vi "Lab Panel V4.85.vi"() -> ()   [LabVIEW 2013] (continued)
          n209 = property on="Tab Control 2" class="TabCtl (strict)"("DisabledEnum"=T14."Enabled" ("Disabled")) -> ()  [unwired: 2 in, 2 out]
          n210 = property on="Tab Control 2" class="TabCtl (strict)"("Value"=0) -> ()  [unwired: 2 in, 2 out]
        }
        frame #9 {
          # "check network directory valid"
          n211 = while {
            stop <- w259 continue-if-true
            w257 = TRUE
            n212 = local read "Network Directory"() -> (w261:path)
            n213 = property on="Tab Control 2" class="TabCtl (strict)"("Value"=5) -> ()  [unwired: 2 in, 2 out]
            n214 = File/Directory Info(path=w261) -> (error out=w262:errorcluster)  [unwired: 1 in, 6 out]
            n215 = Unbundle(w262) -> ("status"=w259:bool)  [unwired: 2 out]
            n216 = case shown="True" w259 {
              frame False {
                n217 = local write "Message"("") -> ()
              }
              frame True {
                "Message" <- "NETWORK DIRECTORY NOT FOUND!!!!"
              }
            }
            n218 = property on="Message" class="Str"("Text.TextColor"=u32 16711680) -> ()  [unwired: 2 in, 2 out]
            n219 = property on="Network Directory" class="Path"("Blinking"=w257) -> ()  [unwired: 2 in, 2 out]
            n220 = property on="Message" class="Str"("Blinking"=w257) -> ()  [unwired: 2 in, 2 out]
          }
        }
        frame #10 {
          w265 = FALSE
          n221 = property on="Message" class="Str"("Blinking"=w265) -> ()  [unwired: 2 in, 2 out]
          n222 = property on="Network Directory" class="Path"("Blinking"=w265) -> ()  [unwired: 2 in, 2 out]
          n223 = property on="Tab Control 2" class="TabCtl (strict)"("Value"=0) -> ()  [unwired: 2 in, 2 out]
        }
      }
    }
    frame #2 {
      n224 = node-c288("loop  delay(mS)") -> (w269:T15)  [unwired: 3 in]
      n225 = timed-loop {
        timing: w269 -> [_]
        timing-out: [_] -> w268
        i -> [w291]
        stop <- "stop" stop-if-true
        n226 = node-c288() -> ()  [unwired: 1 in, 1 out]
        n227 = global write "Global display 1.vi" "stop disp"("stop") -> ()
        n228 = local read "SELECT LAB05-2"() -> (w271:T3)
        n229 = local read "SELECT LAB05-1"() -> (w272:T3)
        n230 = local read "SELECT LAB04-2"() -> (w273:T3)
        n231 = local read "SELECT LAB03-1"() -> (w276:T3)
        n232 = local read "SELECT LAB02-2"() -> (w277:T3)
        n233 = local read "SELECT LAB01-1"() -> (w280:T3)
        n234 = local read "SELECT LAB03-2"() -> (w275:T3)
        n235 = local read "SELECT LAB01-2"() -> (w279:T3)
        n236 = local read "SELECT LAB04-1"() -> (w274:T3)
        n237 = local read "SELECT LAB02-1"() -> (w278:T3)
        n238 = local read "run lab03-2"() -> (w285:bool)
        n239 = local read "run lab04-1"() -> (w284:bool)
        n240 = local read "run lab05-1"() -> (w282:bool)
        n241 = local read "run lab04-2"() -> (w283:bool)
        n242 = local read "run lab05-2"() -> (w281:bool)
        n243 = local read "run lab03-1"() -> (w286:bool)
        n244 = local read "run lab02-2"() -> (w287:bool)
        n245 = local read "run lab02-1"() -> (w288:bool)
        n246 = local read "run lab01-1"() -> (w290:bool)
        n247 = local read "run lab01-2"() -> (w289:bool)
        n248 = stacked-sequence {
          seq-local: [_ w353 _ _ _ _ _ _ _ _ _ _ _ _ _ _ _ _ _ _ _ _] -> [_ _ _ _ _ w2145 _ _ _ _ _ _ _ _ _ _ _ _ _ _ _ _]
          seq-local: [_ w352 _ _ _ _ _ _ _ _ _ _ _ _ _ _ _ _ _ _ _ _] -> [_ _ _ _ _ w2144 _ _ _ _ _ _ _ _ _ _ _ _ _ _ _ _]
          seq-local: [_ w339 _ _ _ _ _ _ _ _ _ _ _ _ _ _ _ _ _ _ _ _] -> [_ _ _ _ _ w2143 _ _ _ _ _ _ _ _ _ _ _ _ _ _ _ _]
          seq-local: [_ w338 _ _ _ _ _ _ _ _ _ _ _ _ _ _ _ _ _ _ _ _] -> [_ _ _ _ _ w2142 _ _ _ _ _ _ _ _ _ _ _ _ _ _ _ _]
          seq-local: [_ w337 _ _ _ _ _ _ _ _ _ _ _ _ _ _ _ _ _ _ _ _] -> [_ _ _ _ _ w2141 _ _ _ _ _ _ _ _ _ _ _ _ _ _ _ _]
          seq-local: [_ w336 _ _ _ _ _ _ _ _ _ _ _ _ _ _ _ _ _ _ _ _] -> [_ _ _ _ _ w2140 _ _ _ _ _ _ _ _ _ _ _ _ _ _ _ _]
          seq-local: [_ w335 _ _ _ _ _ _ _ _ _ _ _ _ _ _ _ _ _ _ _ _] -> [_ _ _ _ _ w2139 _ _ _ _ _ _ _ _ _ _ _ _ _ _ _ _]
          seq-local: [_ w334 _ _ _ _ _ _ _ _ _ _ _ _ _ _ _ _ _ _ _ _] -> [_ _ _ _ _ w2138 _ _ _ _ _ _ _ _ _ _ _ _ _ _ _ _]
          seq-local: [_ w333 _ _ _ _ _ _ _ _ _ _ _ _ _ _ _ _ _ _ _ _] -> [_ _ _ _ _ w2137 _ _ _ _ _ _ _ _ _ _ _ _ _ _ _ _]
          seq-local: [_ w332 _ _ _ _ _ _ _ _ _ _ _ _ _ _ _ _ _ _ _ _] -> [_ _ _ _ _ w2136 _ _ _ _ _ _ _ _ _ _ _ _ _ _ _ _]
          tunnel: w290 -> [_ _ w369 w611 w1735 w2165 w2480 w2967 _ _ _ _ w3371 _ w4305 _ _ w4590 w4893 w5074 _ _]
          tunnel: w289 -> [_ _ w368 w609 w1734 w2164 w2481 w2966 _ _ _ _ w3370 _ w4303 _ _ w4589 w4892 w5072 _ _]
          tunnel: w288 -> [_ _ w367 w607 w1733 w2163 w2479 w2965 _ _ _ _ w3369 _ w4301 _ _ w4588 w4891 w5071 _ _]
          tunnel: w287 -> [_ _ w366 w605 w1732 w2162 w2478 w2964 _ _ _ _ w3368 _ w4299 _ _ w4587 w4890 w5070 _ _]
          tunnel: w286 -> [_ _ w365 w603 w1731 w2161 w2477 w2963 _ _ _ _ w3367 _ w4297 _ _ w4586 w4889 w5069 _ _]
          tunnel: w285 -> [_ _ w364 w601 w1730 w2160 w2476 w2962 _ _ _ _ w3366 _ w4295 _ _ w4585 w4888 w5068 _ _]
          tunnel: w284 -> [_ _ w363 w599 w1729 w2159 w2475 w2961 _ _ _ _ w3365 _ w4293 _ _ w4584 w4887 w5067 _ _]
          tunnel: w283 -> [_ _ w362 w597 w1728 w2158 w2474 w2960 _ _ _ _ w3364 _ w4291 _ _ w4583 w4886 w5066 _ _]
          tunnel: w282 -> [_ _ w361 w595 w1727 w2157 w2473 w2959 _ _ _ _ w3363 _ w4289 _ _ w4582 w4885 w5065 _ _]
          tunnel: w281 -> [_ _ w360 w593 w1726 w2156 w2472 w2958 _ _ _ _ w3362 _ w4287 _ _ w4581 w4884 w5064 _ _]
          tunnel: w280 -> [_ _ _ w610 w1725 w2155 _ _ _ _ _ _ _ _ w4307 _ _ _ _ _ w5368 _]
          tunnel: w279 -> [_ _ _ w608 w1724 w2154 _ _ _ _ _ _ _ _ w4302 _ _ _ _ _ w5367 _]
          tunnel: w278 -> [_ _ _ w606 w1723 w2153 _ _ _ _ _ _ _ _ w4300 _ _ _ _ _ w5366 _]
          tunnel: w277 -> [_ _ _ w604 w1722 w2152 _ _ _ _ _ _ _ _ w4298 _ _ _ _ _ w5365 _]
          tunnel: w276 -> [_ _ _ w602 w1721 w2151 _ _ _ _ _ _ _ _ w4296 _ _ _ _ _ w5364 _]
          tunnel: w275 -> [_ _ _ w600 w1720 w2150 _ _ _ _ _ _ _ _ w4294 _ _ _ _ _ w5363 _]
          tunnel: w274 -> [_ _ _ w598 w1719 w2149 _ _ _ _ _ _ _ _ w4292 _ _ _ _ _ w5362 _]
          tunnel: w273 -> [_ _ _ w596 w1718 w2148 _ _ _ _ _ _ _ _ w4290 _ _ _ _ _ w5361 _]
          tunnel: w272 -> [_ _ _ w594 w1717 w2147 _ _ _ _ _ _ _ _ w4288 _ _ _ _ _ w5360 _]
          tunnel: w271 -> [_ _ _ w592 w1716 w2146 _ _ _ _ _ _ _ _ w4286 _ _ _ _ _ w5359 _]
          frame #0 {
            w295 = FALSE
            w300 = 0.5
            # "set up cycle control"
            n249 = local read "jig cycle"() -> (w299:dbl)
            n250 = Divide(x="JIG ON TIME (S)", y=w300) -> (x/y=→"on loops":dbl)
            n251 = Divide(x="JIG OFF TIME (S)", y=w300) -> (x/y=→"off loops":dbl)
            n252 = Increment(x=w299) -> (x+1=w298:dbl)
            n253 = local write "TEMP"(w295) -> ()
            n254 = local write "AI"(w295) -> ()
            n255 = local write "jig cycle"(w298) -> ()
            n256 = event shown="[1] \"ADMIN\": Value Change" {
              selector: _ -> [_ _]
              dyn-events: _ -> [_ _]
              timeout: 10 -> [_ _]
              event Timeout {
                n257 = event-data() -> ()  [unwired: 1 in, 3 out]
              }
              event "ADMIN": Value Change {
                n258 = event-data() -> ()  [unwired: 1 in, 6 out]
                n259 = stacked-sequence {
                  seq-local: [_ w304 _] -> [_ _ w305]
                  frame #0 {
                    n260 = global write "Global 1.vi" "password"("9999") -> ()
                  }
                  frame #1 {
                    n261 = call "sub vi - password 1.vi"() -> ("RESULT"=w304:bool)  [unwired: 11 in]
                  }
                  frame #2 {
                    w307 = FALSE
                    n262 = property on="Tab Control 2" class="TabCtl (strict)"() -> ("Pages"=w311:refnum<vi>[])  [unwired: 2 in, 2 out]
                    n263 = Select(t=TRUE, s=w305, f=w307) -> (s? t:f=w306:bool)
                    n264 = Index Array(array=w311, index=9) -> (element=w309:refnum<vi>)
                    n265 = property class="Page"(reference=w309, "PageVis"=w306) -> ()  [unwired: 1 in, 2 out]
                    n266 = local write "ADMIN"(w307) -> ()
                  }
                }
              }
            }
          }
          frame #1 {
            w349 = 60.0
            # "convert temperature rise minutes to cycles"
            n267 = local read "SET LAB05-2"() -> (w313:T5)
            n268 = local read "SET LAB05-1"() -> (w315:T5)
            n269 = local read "SET LAB04-2"() -> (w317:T5)
            n270 = local read "SET LAB01-1"() -> (w331:T5)
            n271 = local read "SET LAB01-2"() -> (w329:T5)
            n272 = local read "SET LAB02-2"() -> (w325:T5)
            n273 = local read "SET LAB04-1"() -> (w319:T5)
            n274 = local read "SET LAB03-1"() -> (w323:T5)
            n275 = local read "SET LAB03-2"() -> (w321:T5)
            n276 = local read "SET LAB02-1"() -> (w327:T5)
            n277 = local read "JIG OFF TIME (S)"() -> (w354:dbl)
            n278 = local read "JIG ON TIME (S)"() -> (w355:dbl)
            n279 = Unbundle(w313) -> ("T-RISE mins"=w312:dbl)  [unwired: 4 out]
            n280 = Unbundle(w315) -> ("T-RISE mins"=w314:dbl)  [unwired: 4 out]
            n281 = Unbundle(w331) -> ("T-RISE mins"=w330:dbl)  [unwired: 4 out]
            n282 = Unbundle(w317) -> ("T-RISE mins"=w316:dbl)  [unwired: 4 out]
            n283 = Unbundle(w329) -> ("T-RISE mins"=w328:dbl)  [unwired: 4 out]
            n284 = Unbundle(w327) -> ("T-RISE mins"=w326:dbl)  [unwired: 4 out]
            n285 = Unbundle(w319) -> ("T-RISE mins"=w318:dbl)  [unwired: 4 out]
            n286 = Unbundle(w325) -> ("T-RISE mins"=w324:dbl)  [unwired: 4 out]
            n287 = Unbundle(w321) -> ("T-RISE mins"=w320:dbl)  [unwired: 4 out]
            n288 = Unbundle(w323) -> ("T-RISE mins"=w322:dbl)  [unwired: 4 out]
            n289 = Add(x=w355, y=w354) -> (x+y=w348:dbl)
            n290 = Multiply(x=w349, y=w320) -> (x*y=w344:dbl)
            n291 = Multiply(x=w349, y=w318) -> (x*y=w343:dbl)
            n292 = Multiply(x=w349, y=w316) -> (x*y=w342:dbl)
            n293 = Multiply(x=w349, y=w314) -> (x*y=w341:dbl)
            n294 = Multiply(x=w349, y=w312) -> (x*y=w340:dbl)
            n295 = Multiply(x=w349, y=w328) -> (x*y=w350:dbl)
            n296 = Multiply(x=w349, y=w322) -> (x*y=w345:dbl)
            n297 = Multiply(x=w349, y=w330) -> (x*y=w351:dbl)
            n298 = Multiply(x=w349, y=w326) -> (x*y=w347:dbl)
            n299 = Multiply(x=w349, y=w324) -> (x*y=w346:dbl)
            n300 = Divide(x=w341, y=w348) -> (x/y=w333:dbl)
            n301 = Divide(x=w342, y=w348) -> (x/y=w334:dbl)
            n302 = Divide(x=w343, y=w348) -> (x/y=w335:dbl)
            n303 = Divide(x=w340, y=w348) -> (x/y=w332:dbl)
            n304 = Divide(x=w345, y=w348) -> (x/y=w337:dbl)
            n305 = Divide(x=w351, y=w348) -> (x/y=w353:dbl)
            n306 = Divide(x=w350, y=w348) -> (x/y=w352:dbl)
            n307 = Divide(x=w347, y=w348) -> (x/y=w339:dbl)
            n308 = Divide(x=w346, y=w348) -> (x/y=w338:dbl)
            n309 = Divide(x=w344, y=w348) -> (x/y=w336:dbl)
          }
          frame #2 {
            # "control cycle loops"
            n310 = local read "JIG OFF TIME (S)"() -> (w358:dbl)
            n311 = local read "JIG ON TIME (S)"() -> (w357:dbl)
            n312 = local read "jig cycle"() -> (w371:dbl)
            n313 = local read "on loops"() -> (w373:dbl)
            n314 = local read "off loops"() -> (w372:dbl)
            n315 = Add(x=w358, y=w357) -> (x+y=w356:dbl)
            n316 = Add(x=w373, y=w372) -> (x+y=w359:dbl)
            n317 = Greater Or Equal?(x=w371, y=w359) -> (x >= y?=w370:bool)
            n318 = case shown="True" w370 {
              tunnel: w369 -> [_ w408]
              tunnel: w368 -> [_ w407]
              tunnel: w367 -> [_ w406]
              tunnel: w366 -> [_ w405]
              tunnel: w365 -> [_ w404]
              tunnel: w364 -> [_ w403]
              tunnel: w363 -> [_ w402]
              tunnel: w362 -> [_ w401]
              tunnel: w361 -> [_ w400]
              tunnel: w360 -> [_ w399]
              tunnel: w356 -> [_ w398]
              frame False {
              }
              frame True {
                # "increment cycle value and convert cycles to minutes for temp rise"
                n319 = local read "Temp Loops"() -> (w375:dbl)
                n320 = local read "JIG RELAY CYCLES"() -> (w397:T7)
                n321 = Increment(x=w375) -> (x+1=w374:dbl)
                n322 = local write "Temp Loops"(w374) -> ()
                n323 = Unbundle By Name(w397) -> ("LAB01-1"=w395:dbl, "LAB01-2"=w393:dbl, "LAB02-1"=w391:dbl, "LAB02-2"=w389:dbl, "LAB03-1"=w387:dbl, "LAB03-2"=w385:dbl, "LAB04-1"=w383:dbl, "LAB04-2"=w381:dbl, "LAB05-1"=w379:dbl, "LAB05-2"=w377:dbl)
                n324 = stacked-sequence {
                  tunnel: w408 -> [w420 _ _ _ _ _ _ _ _ _]
                  tunnel: w407 -> [_ w437 _ _ _ _ _ _ _ _]
                  tunnel: w406 -> [_ _ w454 _ _ _ _ _ _ _]
                  tunnel: w405 -> [_ _ _ w471 _ _ _ _ _ _]
                  tunnel: w404 -> [_ _ _ _ w488 _ _ _ _ _]
                  tunnel: w403 -> [_ _ _ _ _ w505 _ _ _ _]
                  tunnel: w402 -> [_ _ _ _ _ _ w522 _ _ _]
                  tunnel: w401 -> [_ _ _ _ _ _ _ w539 _ _]
                  tunnel: w400 -> [_ _ _ _ _ _ _ _ w556 _]
                  tunnel: w399 -> [_ _ _ _ _ _ _ _ _ w573]
                  tunnel: w398 -> [w417 w434 w451 w468 w485 w502 w519 w536 w553 w570]
                  tunnel: w395 -> [w411 _ _ _ _ _ _ _ _ _]
                  tunnel: [w410 _ _ _ _ _ _ _ _ _] -> w394
                  tunnel: w393 -> [_ w428 _ _ _ _ _ _ _ _]
                  tunnel: [_ w427 _ _ _ _ _ _ _ _] -> w392
                  tunnel: w391 -> [_ _ w445 _ _ _ _ _ _ _]
                  tunnel: [_ _ w444 _ _ _ _ _ _ _] -> w390
                  tunnel: w389 -> [_ _ _ w462 _ _ _ _ _ _]
                  tunnel: [_ _ _ w461 _ _ _ _ _ _] -> w388
                  tunnel: w387 -> [_ _ _ _ w479 _ _ _ _ _]
                  tunnel: [_ _ _ _ w478 _ _ _ _ _] -> w386
                  tunnel: w385 -> [_ _ _ _ _ w496 _ _ _ _]
                  tunnel: [_ _ _ _ _ w495 _ _ _ _] -> w384
                  tunnel: w383 -> [_ _ _ _ _ _ w513 _ _ _]
                  tunnel: [_ _ _ _ _ _ w512 _ _ _] -> w382
                  tunnel: w381 -> [_ _ _ _ _ _ _ w530 _ _]
                  tunnel: [_ _ _ _ _ _ _ w529 _ _] -> w380
                  tunnel: w379 -> [_ _ _ _ _ _ _ _ w547 _]
                  tunnel: [_ _ _ _ _ _ _ _ w546 _] -> w378
                  tunnel: w377 -> [_ _ _ _ _ _ _ _ _ w564]
                  tunnel: [_ _ _ _ _ _ _ _ _ w563] -> w376
                  frame #0 {
                    n325 = local read "DISP LAB01-1"() -> (w415:T4)
                    n326 = Unbundle(w415) -> ("CYCLE"=w416:dbl)  [unwired: 2 out]
                    n327 = case shown="True" w420 {
                      tunnel: w416 -> [w422 w426]
                      tunnel: [w422 w425] -> w414
                      tunnel: w411 -> [w421 w424]
                      tunnel: [w421 w423] -> w410
                      frame False {
                      }
                      frame True {
                        n328 = Increment(x=w424) -> (x+1=w423:dbl)
                        n329 = Increment(x=w426) -> (x+1=w425:dbl)
                      }
                    }
                    n330 = Multiply(x=w414, y=w417) -> (x*y=w418:dbl)
                    n331 = Divide(x=w418, y=60.0) -> (x/y=w413:dbl)
                    n332 = Bundle(cluster=w415, "CYCLE"=w414, "MINS"=w413) -> (w412:T4)  [unwired: 1 in]
                    n333 = local write "DISP LAB01-1"(w412) -> ()
                  }
                  frame #1 {
                    n334 = local read "DISP LAB01-2"() -> (w432:T4)
                    n335 = Unbundle(w432) -> ("CYCLE"=w433:dbl)  [unwired: 2 out]
                    n336 = case shown="True" w437 {
                      tunnel: w433 -> [w439 w443]
                      tunnel: [w439 w442] -> w430
                      tunnel: w428 -> [w438 w441]
                      tunnel: [w438 w440] -> w427
                      frame False {
                      }
                      frame True {
                        n337 = Increment(x=w441) -> (x+1=w440:dbl)
                        n338 = Increment(x=w443) -> (x+1=w442:dbl)
                      }
                    }
                    n339 = Multiply(x=w430, y=w434) -> (x*y=w435:dbl)
                    n340 = Divide(x=w435, y=60.0) -> (x/y=w429:dbl)
                    n341 = Bundle(cluster=w432, "CYCLE"=w430, "MINS"=w429) -> (w431:T4)  [unwired: 1 in]
                    n342 = local write "DISP LAB01-2"(w431) -> ()
                  }
                  frame #2 {
                    n343 = local read "DISP LAB02-1"() -> (w449:T4)
                    n344 = Unbundle(w449) -> ("CYCLE"=w450:dbl)  [unwired: 2 out]
                    n345 = case shown="True" w454 {
                      tunnel: [w456 w460] -> w447
                      tunnel: w450 -> [w456 w459]
                      tunnel: w445 -> [w455 w458]
                      tunnel: [w455 w457] -> w444
                      frame False {
                      }
                      frame True {
                        n346 = Increment(x=w458) -> (x+1=w457:dbl)
                        n347 = Increment(x=w459) -> (x+1=w460:dbl)
                      }
                    }
                    n348 = Multiply(x=w447, y=w451) -> (x*y=w452:dbl)
                    n349 = Divide(x=w452, y=60.0) -> (x/y=w446:dbl)
                    n350 = Bundle(cluster=w449, "CYCLE"=w447, "MINS"=w446) -> (w448:T4)  [unwired: 1 in]
                    n351 = local write "DISP LAB02-1"(w448) -> ()
                  }
                  frame #3 {
                    n352 = local read "DISP LAB02-2"() -> (w466:T4)
                    n353 = Unbundle(w466) -> ("CYCLE"=w467:dbl)  [unwired: 2 out]
                    n354 = case shown="True" w471 {
                      tunnel: [w473 w477] -> w465
                      tunnel: w467 -> [w473 w476]
                      tunnel: w462 -> [w472 w475]
                      tunnel: [w472 w474] -> w461
                      frame False {
                      }
                      frame True {
                        n355 = Increment(x=w475) -> (x+1=w474:dbl)
                        n356 = Increment(x=w476) -> (x+1=w477:dbl)
                      }
                    }
                    n357 = Multiply(x=w465, y=w468) -> (x*y=w469:dbl)
                    n358 = Divide(x=w469, y=60.0) -> (x/y=w464:dbl)
                    n359 = Bundle(cluster=w466, "CYCLE"=w465, "MINS"=w464) -> (w463:T4)  [unwired: 1 in]
                    n360 = local write "DISP LAB02-2"(w463) -> ()
                  }
                  frame #4 {
                    n361 = local read "DISP LAB03-1"() -> (w483:T4)
                    n362 = Unbundle(w483) -> ("CYCLE"=w484:dbl)  [unwired: 2 out]
                    n363 = case shown="True" w488 {
                      tunnel: [w490 w494] -> w480
                      tunnel: w484 -> [w490 w493]
                      tunnel: w479 -> [w489 w492]
                      tunnel: [w489 w491] -> w478
                      frame False {
                      }
                      frame True {
                        n364 = Increment(x=w492) -> (x+1=w491:dbl)
                        n365 = Increment(x=w493) -> (x+1=w494:dbl)
                      }
                    }
                    n366 = Multiply(x=w480, y=w485) -> (x*y=w486:dbl)
                    n367 = Divide(x=w486, y=60.0) -> (x/y=w481:dbl)
                    n368 = Bundle(cluster=w483, "CYCLE"=w480, "MINS"=w481) -> (w482:T4)  [unwired: 1 in]
                    n369 = local write "DISP LAB03-1"(w482) -> ()
                  }
                  frame #5 {
                    n370 = local read "DISP LAB03-2"() -> (w500:T4)
                    n371 = Unbundle(w500) -> ("CYCLE"=w501:dbl)  [unwired: 2 out]
                    n372 = case shown="True" w505 {
                      tunnel: [w507 w511] -> w499
                      tunnel: w501 -> [w507 w510]
                      tunnel: w496 -> [w506 w509]
                      tunnel: [w506 w508] -> w495
                      frame False {
                      }
                      frame True {
                        n373 = Increment(x=w509) -> (x+1=w508:dbl)
                        n374 = Increment(x=w510) -> (x+1=w511:dbl)
                      }
                    }
                    n375 = Multiply(x=w499, y=w502) -> (x*y=w503:dbl)
                    n376 = Divide(x=w503, y=60.0) -> (x/y=w498:dbl)
                    n377 = Bundle(cluster=w500, "CYCLE"=w499, "MINS"=w498) -> (w497:T4)  [unwired: 1 in]
                    n378 = local write "DISP LAB03-2"(w497) -> ()
                  }
                  frame #6 {
                    n379 = local read "DISP LAB04-1"() -> (w517:T4)
                    n380 = Unbundle(w517) -> ("CYCLE"=w518:dbl)  [unwired: 2 out]
                    n381 = case shown="True" w522 {
                      tunnel: [w524 w528] -> w515
                      tunnel: w518 -> [w524 w527]
                      tunnel: w513 -> [w523 w526]
                      tunnel: [w523 w525] -> w512
                      frame False {
                      }
                      frame True {
                        n382 = Increment(x=w526) -> (x+1=w525:dbl)
                        n383 = Increment(x=w527) -> (x+1=w528:dbl)
                      }
                    }
                    n384 = Multiply(x=w515, y=w519) -> (x*y=w520:dbl)
                    n385 = Divide(x=w520, y=60.0) -> (x/y=w514:dbl)
                    n386 = Bundle(cluster=w517, "CYCLE"=w515, "MINS"=w514) -> (w516:T4)  [unwired: 1 in]
                    n387 = local write "DISP LAB04-1"(w516) -> ()
                  }
                  frame #7 {
                    n388 = local read "DISP LAB04-2"() -> (w534:T4)
                    n389 = Unbundle(w534) -> ("CYCLE"=w535:dbl)  [unwired: 2 out]
                    n390 = case shown="True" w539 {
                      tunnel: [w541 w545] -> w532
                      tunnel: w535 -> [w541 w544]
                      tunnel: w530 -> [w540 w543]
                      tunnel: [w540 w542] -> w529
                      frame False {
                      }
                      frame True {
                        n391 = Increment(x=w543) -> (x+1=w542:dbl)
                        n392 = Increment(x=w544) -> (x+1=w545:dbl)
                      }
                    }
                    n393 = Multiply(x=w532, y=w536) -> (x*y=w538:dbl)
                    n394 = Divide(x=w538, y=60.0) -> (x/y=w531:dbl)
                    n395 = Bundle(cluster=w534, "CYCLE"=w532, "MINS"=w531) -> (w533:T4)  [unwired: 1 in]
                    n396 = local write "DISP LAB04-2"(w533) -> ()
                  }
                  frame #8 {
                    n397 = local read "DISP LAB05-1"() -> (w551:T4)
                    n398 = Unbundle(w551) -> ("CYCLE"=w552:dbl)  [unwired: 2 out]
                    n399 = case shown="True" w556 {
                      tunnel: [w558 w562] -> w549
                      tunnel: w552 -> [w558 w561]
                      tunnel: w547 -> [w557 w560]
                      tunnel: [w557 w559] -> w546
                      frame False {
                      }
                      frame True {
                        n400 = Increment(x=w560) -> (x+1=w559:dbl)
                        n401 = Increment(x=w561) -> (x+1=w562:dbl)
                      }
                    }
                    n402 = Multiply(x=w549, y=w553) -> (x*y=w554:dbl)
                    n403 = Divide(x=w554, y=60.0) -> (x/y=w548:dbl)
                    n404 = Bundle(cluster=w551, "CYCLE"=w549, "MINS"=w548) -> (w550:T4)  [unwired: 1 in]
                    n405 = local write "DISP LAB05-1"(w550) -> ()
                  }
                  frame #9 {
                    n406 = local read "DISP LAB05-2"() -> (w569:T4)
                    n407 = Unbundle(w569) -> ("CYCLE"=w568:dbl)  [unwired: 2 out]
                    n408 = case shown="True" w573 {
                      tunnel: [w575 w579] -> w567
                      tunnel: w568 -> [w575 w578]
                      tunnel: w564 -> [w574 w577]
                      tunnel: [w574 w576] -> w563
                      frame False {
                      }
                      frame True {
                        n409 = Increment(x=w577) -> (x+1=w576:dbl)
                        n410 = Increment(x=w578) -> (x+1=w579:dbl)
                      }
                    }
                    n411 = Multiply(x=w567, y=w570) -> (x*y=w571:dbl)
                    n412 = Divide(x=w571, y=60.0) -> (x/y=w566:dbl)
                    n413 = Bundle(cluster=w569, "CYCLE"=w567, "MINS"=w566) -> (w565:T4)  [unwired: 1 in]
                    n414 = local write "DISP LAB05-2"(w565) -> ()
                  }
                }
                n415 = local write "jig cycle"(0) -> ()
                n416 = Bundle By Name(cluster=w397, "LAB01-1"=w394, "LAB01-2"=w392, "LAB02-1"=w390, "LAB02-2"=w388, "LAB03-1"=w386, "LAB03-2"=w384, "LAB04-1"=w382, "LAB04-2"=w380, "LAB05-1"=w378, "LAB05-2"=w376) -> (w396:T7)
                n417 = local write "JIG RELAY CYCLES"(w396) -> ()
              }
            }
          }
          frame #3 {
            # "START & STOP test RUN switch change, start test if true and stop test if false"
            n418 = Get Date/Time In Seconds() -> (seconds since 1Jan1904=w590:timestamp)
            n419 = local read "C drive data root dir"() -> (w583:path)
            n420 = Format Date/Time String(time format string (%c)="%b\\%a%d", seconds (now)=w590) -> (date/time string=w614:string)  [unwired: 1 in]
            n421 = Format Date/Time String(time format string (%c)="%H%M", seconds (now)=w590) -> (date/time string=w612:string)  [unwired: 1 in]
            n422 = Format Date/Time String(time format string (%c)="LabPanel%Y", seconds (now)=w590) -> (date/time string=w589:string)  [unwired: 1 in]
            n423 = Path To String(path=w583) -> (string=w586:string)
            n424 = global write "Global 1.vi" "C drive root path"(w583) -> ()
            n425 = Concatenate Strings(w586, "\\") -> (w584:string)
            n426 = event shown="[1] \"RUN LAB01-1\": Value Change" {
              selector: _ -> [_ _ _ _ _ _ _ _ _ _ _]
              dyn-events: _ -> [_ _ _ _ _ _ _ _ _ _ _]
              timeout: 10 -> [_ _ _ _ _ _ _ _ _ _ _]
              tunnel: w584 -> [_ w625 w735 w845 w955 w1065 w1175 w1285 w1395 w1505 w1615]
              tunnel: w614 -> [_ w624 w734 w844 w954 w1064 w1174 w1284 w1394 w1504 w1614]
              tunnel: w612 -> [_ w622 w733 w843 w953 w1063 w1173 w1283 w1393 w1503 w1613]
              tunnel: w610 -> [_ w623 _ _ _ _ _ _ _ _ _]
              tunnel: w611 -> [_ _ _ _ _ _ _ _ _ _ _]
              tunnel: w609 -> [_ _ _ _ _ _ _ _ _ _ _]
              tunnel: w608 -> [_ _ w732 _ _ _ _ _ _ _ _]
              tunnel: w607 -> [_ _ _ _ _ _ _ _ _ _ _]
              tunnel: w606 -> [_ _ _ w842 _ _ _ _ _ _ _]
              tunnel: w605 -> [_ _ _ _ _ _ _ _ _ _ _]
              tunnel: w604 -> [_ _ _ _ w952 _ _ _ _ _ _]
              tunnel: w603 -> [_ _ _ _ _ _ _ _ _ _ _]
              tunnel: w602 -> [_ _ _ _ _ w1062 _ _ _ _ _]
              tunnel: w601 -> [_ _ _ _ _ _ _ _ _ _ _]
              tunnel: w600 -> [_ _ _ _ _ _ w1172 _ _ _ _]
              tunnel: w599 -> [_ _ _ _ _ _ _ _ _ _ _]
              tunnel: w598 -> [_ _ _ _ _ _ _ w1282 _ _ _]
              tunnel: w597 -> [_ _ _ _ _ _ _ _ _ _ _]
              tunnel: w596 -> [_ _ _ _ _ _ _ _ w1392 _ _]
              tunnel: w595 -> [_ _ _ _ _ _ _ _ _ _ _]
              tunnel: w594 -> [_ _ _ _ _ _ _ _ _ w1502 _]
              tunnel: w593 -> [_ _ _ _ _ _ _ _ _ _ _]
              tunnel: w592 -> [_ _ _ _ _ _ _ _ _ _ w1612]
              tunnel: w589 -> [_ w621 w731 w841 w951 w1061 w1171 w1281 w1391 w1501 w1611]
              tunnel: [_ w620 w730 w840 w950 w1060 w1170 w1280 w1390 w1500 w1610] -> w587
              tunnel: "RESET CYCLES TO ZERO?" -> [_ w618 w728 w838 w948 w1058 w1168 w1278 w1388 w1498 w1608]
              tunnel: "YES" -> [_ w617 w727 w837 w947 w1057 w1167 w1277 w1387 w1497 w1607]
              tunnel: "NO" -> [_ w616 w726 w836 w946 w1056 w1166 w1276 w1386 w1496 w1606]
              event Timeout {
                n427 = event-data() -> ()  [unwired: 1 in, 3 out]
              }
              event "RUN LAB01-1": Value Change {
                n428 = event-data() -> ("NewVal"=w619:bool)  [unwired: 1 in, 5 out]
                n429 = local write "run lab01-1"(w619) -> ()
                n430 = case shown="True" w619 {
                  tunnel: w625 -> [_ w661]
                  tunnel: w624 -> [_ w660]
                  tunnel: w623 -> [w627 w659]
                  tunnel: w622 -> [_ w658]
                  tunnel: w621 -> [_ w657]
                  tunnel: [w626 w656] -> w620
                  tunnel: w618 -> [_ w655]
                  tunnel: w617 -> [_ w654]
                  tunnel: w616 -> [_ w653]
                  frame False {
                    # "stop test"
                    n431 = stacked-sequence {
                      tunnel: w627 -> [_ w639 _]
                      tunnel: [_ w631 _] -> w626
                      frame #0 {
                        n432 = local read "DISP LAB01-1"() -> (w630:T4)
                        n433 = Bundle(cluster=w630, "STATUS"="STOP") -> (w628:T4)  [unwired: 2 in]
                        n434 = local write "DISP LAB01-1"(w628) -> ()
                      }
                      frame #1 {
                        n435 = local read "DISP LAB01-1"() -> (w638:T4)
                        n436 = Unbundle(w638) -> ("CYCLE"=w636:dbl, "MINS"=w637:dbl)  [unwired: 1 out]
                        n437 = case shown="\"CYCLE TEST\"" w639 {
                          tunnel: w637 -> [_ _ w646]
                          tunnel: w636 -> [w644 w645 _]
                          tunnel: [w644 w645 w646] -> w635
                          frame "CHART TEST", Default {
                          }
                          frame "CYCLE TEST" {
                          }
                          frame "T-RISE TEST" {
                          }
                        }
                        n438 = local read "TDMS LAB01-1"() -> (w643:refnum<k34>)
                        n439 = Build Array("STOPPED") -> (w640:string[])
                        n440 = Build Array(w635) -> (w634:dbl[])
                        n441 = TDMS Write(0:w643, 5:"TEST RESULT", 7:w640, 9:w634) -> (4:w632:refnum<k34>, 15:w633:errorcluster)  [unwired: 2 in, 2 out]
                        n442 = TDMS Close(8:w633, 11:w632) -> (0:w631:errorcluster)  [unwired: 1 out]
                      }
                      frame #2 {
                        n443 = stacked-sequence {
                          tunnel: "LAB01-1" -> [w649 w651]
                          frame #0 {
                            n444 = call "sub vi - defrag tdms v1.vi"("panel id"=w649) -> ("error out"=w648:errorcluster)  [unwired: 10 in]
                            n445 = local write "data file error"(w648) -> ()
                          }
                          frame #1 {
                            n446 = call "Save data file to network drive v2.vi"("panel id"=w651) -> ("network file save error"=w650:errorcluster)  [unwired: 9 in, 1 out]
                            n447 = local write "RESULT LAB01-1"(FALSE) -> ()
                            n448 = local write "data file error"(w650) -> ()
                          }
                        }
                      }
                    }
                  }
                  frame True {
                    # "start new test and create test file"
                    n449 = stacked-sequence {
                      seq-local: [w662 _ _ _ _] -> [_ w683 _ _ _]
                      tunnel: w661 -> [w667 _ _ _ _]
                      tunnel: w660 -> [w663 _ _ _ _]
                      tunnel: w659 -> [w677 _ _ _ _]
                      tunnel: w658 -> [w670 _ _ _ _]
                      tunnel: w657 -> [w665 _ _ _ _]
                      tunnel: [_ w684 _ _ _] -> w656
                      tunnel: w655 -> [_ _ _ w705 _]
                      tunnel: w654 -> [_ _ _ w715 _]
                      tunnel: w653 -> [_ _ _ w714 _]
                      frame #0 {
                        w664 = "\\"
                        n450 = case shown="\"CHART TEST\", Default" w677 {
                          tunnel: ["L01-1-CHART TEST-" "L01-1-CYCLE TEST-" "L01-1-T-RISE TEST-"] -> w673
                          frame "CHART TEST", Default {
                          }
                          frame "CYCLE TEST" {
                          }
                          frame "T-RISE TEST" {
                          }
                        }
                        n451 = local read "SET LAB01-1"() -> (w672:T5)
                        n452 = Unbundle(w672) -> ("DESCRIPTION"=w671:string)  [unwired: 4 out]
                        n453 = Concatenate Strings(w667, "\\", w665, w664, w663, w664) -> (w674:string)
                        n454 = String To Path(string=w674) -> (path=w676:path)
                        n455 = Concatenate Strings(w674, w673, w671, "-", w670, ".tdms") -> (w662:string)
                        n456 = Create Folder(path (use dialog)=w676) -> (error out=w675:errorcluster)  [unwired: 2 in, 2 out]
                        n457 = call <vilib>:"Clear Errors.vi"("error in (no error)"=w675) -> ()  [unwired: 6 in, 1 out]
                        n458 = global write "Global 1.vi" "LAB01-1 FILE"(w662) -> ()
                      }
                      frame #1 {
                        (unwired) FALSE
                        n459 = String To Path(string=w683) -> (path=w681:path)
                        n460 = TDMS Open(6:FALSE, 10:T18."create or replace" ("operation (0:open)"), 11:w681) -> (0:w684:errorcluster, 3:→"TDMS LAB01-1":refnum<k34>)  [unwired: 4 in]
                      }
                      frame #2 {
                        n461 = local read "TDMS LAB01-1"() -> (w703:refnum<k34>)
                        n462 = local read "SET LAB01-1"() -> (w692:T5)
                        n463 = Build Array("Testers Name", "Description", "Set Test Cycles", "T-Rise minutes", "T-Rise Deg C") -> (w693:string[])
                        n464 = Unbundle(w692) -> ("NAME"=w691:string, "DESCRIPTION"=w690:string, "CYCLES"=w689:dbl, "T-RISE mins"=w688:dbl, "T-RISE deg C"=w687:dbl)
                        n465 = Number To Decimal String(number=w689) -> (decimal integer string=w702:string)  [unwired: 1 in]
                        n466 = Number To Decimal String(number=w688) -> (decimal integer string=w701:string)  [unwired: 1 in]
                        n467 = Number To Decimal String(number=w687) -> (decimal integer string=w700:string)  [unwired: 1 in]
                        n468 = Build Array(w691, w690, w702, w701, w700) -> (w699:string[])
                        n469 = TDMS Set Properties(5:w699, 7:w693, 11:w703) -> ()  [unwired: 3 in, 4 out]
                      }
                      frame #3 {
                        n470 = local read "DISP LAB01-1"() -> (w713:T4)
                        n471 = Concatenate Strings("LAB01-1  ", w705) -> (w704:string)
                        n472 = Two Button Dialog(message=w704, 1:w714, 2:w715) -> (T button?=w707:bool)
                        n473 = case shown="True" w707 {
                          tunnel: w713 -> [w718 w719]
                          tunnel: [w718 w719] -> w712
                          tunnel: [w717 w720] -> w711
                          tunnel: [w716 w720] -> w710
                          frame False {
                            n474 = Unbundle(w718) -> ("CYCLE"=w717:dbl, "MINS"=w716:dbl)  [unwired: 1 out]
                          }
                          frame True {
                            w720 = 0.0
                          }
                        }
                        n475 = Bundle(cluster=w712, "CYCLE"=w711, "MINS"=w710, "STATUS"="RUN") -> (w709:T4)
                        n476 = local write "DISP LAB01-1"(w709) -> ()
                      }
                      frame #4 {
                        n477 = local read "SIG LAB01-1"() -> (w723:T2)
                        n478 = local read "TEMP START LAB01-1"() -> (w725:cluster{"TL":dbl, "TN":dbl})
                        n479 = Unbundle(w723) -> ("Tmp Live"=w722:dbl, "Tmp Neut"=w721:dbl)  [unwired: 3 out]
                        n480 = Bundle(cluster=w725, "TL"=w722, "TN"=w721) -> (w724:cluster{"TL":dbl, "TN":dbl})
                        n481 = local write "TEMP START LAB01-1"(w724) -> ()
                      }
                    }
                  }
                }
              }
              event "RUN LAB01-2": Value Change {
                n482 = event-data() -> ("NewVal"=w729:bool)  [unwired: 1 in, 5 out]
                n483 = local write "run lab01-2"(w729) -> ()
                n484 = case shown="True" w729 {
                  tunnel: w735 -> [_ w771]
                  tunnel: w734 -> [_ w770]
                  tunnel: w732 -> [w737 w769]
                  tunnel: w733 -> [_ w768]
                  tunnel: w731 -> [_ w767]
                  tunnel: [w736 w766] -> w730
                  tunnel: w728 -> [_ w765]
                  tunnel: w727 -> [_ w764]
                  tunnel: w726 -> [_ w763]
                  frame False {
                    # "stop test"
                    n485 = stacked-sequence {
                      tunnel: w737 -> [w746 _]
                      tunnel: [w738 _] -> w736
                      frame #0 {
                        n486 = local read "DISP LAB01-2"() -> (w745:T4)
                        n487 = Unbundle(w745) -> ("CYCLE"=w743:dbl, "MINS"=w744:dbl)  [unwired: 1 out]
                        n488 = case shown="\"CHART TEST\", Default" w746 {
                          tunnel: w744 -> [_ _ w753]
                          tunnel: w743 -> [w751 w752 _]
                          tunnel: [w751 w752 w753] -> w742
                          frame "CHART TEST", Default {
                          }
                          frame "CYCLE TEST" {
                          }
                          frame "T-RISE TEST" {
                          }
                        }
                        n489 = local read "TDMS LAB01-2"() -> (w750:refnum<k34>)
                        n490 = Build Array("STOPPED") -> (w747:string[])
                        n491 = Build Array(w742) -> (w741:dbl[])
                        n492 = TDMS Write(0:w750, 5:"TEST RESULT", 7:w747, 9:w741) -> (4:w739:refnum<k34>, 15:w740:errorcluster)  [unwired: 2 in, 2 out]
                        n493 = TDMS Close(8:w740, 11:w739) -> (0:w738:errorcluster)  [unwired: 1 out]
                      }
                      frame #1 {
                        n494 = local read "DISP LAB01-2"() -> (w757:T4)
                        n495 = stacked-sequence {
                          tunnel: "LAB01-2" -> [w759 w761]
                          frame #0 {
                            n496 = call "sub vi - defrag tdms v1.vi"("panel id"=w759) -> ("error out"=w758:errorcluster)  [unwired: 10 in]
                            n497 = local write "data file error"(w758) -> ()
                          }
                          frame #1 {
                            n498 = call "Save data file to network drive v2.vi"("panel id"=w761) -> ("network file save error"=w760:errorcluster)  [unwired: 9 in, 1 out]
                            n499 = local write "RESULT LAB01-2"(FALSE) -> ()
                            n500 = local write "data file error"(w760) -> ()
                          }
                        }
                        n501 = Bundle(cluster=w757, "STATUS"="STOP") -> (w755:T4)  [unwired: 2 in]
                        n502 = local write "DISP LAB01-2"(w755) -> ()
                      }
                    }
                  }
                  frame True {
                    # "start new test and create test file"
                    n503 = stacked-sequence {
                      seq-local: [w772 _ _ _ _] -> [_ w796 _ _ _]
                      tunnel: w771 -> [w777 _ _ _ _]
                      tunnel: w770 -> [w774 _ _ _ _]
                      tunnel: w769 -> [w787 _ _ _ _]
                      tunnel: w768 -> [w780 _ _ _ _]
                      tunnel: w767 -> [w775 _ _ _ _]
                      tunnel: [_ w791 _ _ _] -> w766
                      tunnel: w765 -> [_ _ _ w818 _]
                      tunnel: w764 -> [_ _ _ w817 _]
                      tunnel: w763 -> [_ _ _ w816 _]
                      frame #0 {
                        w773 = "\\"
                        n504 = local read "SET LAB01-2"() -> (w782:T5)
                        n505 = case shown="\"CYCLE TEST\"" w787 {
                          tunnel: ["L01-2-CHART TEST-" "L01-2-CYCLE TEST-" "L01-2-T-RISE TEST-"] -> w783
                          frame "CHART TEST", Default {
                          }
                          frame "CYCLE TEST" {
                          }
                          frame "T-RISE TEST" {
                          }
                        }
                        n506 = Unbundle(w782) -> ("DESCRIPTION"=w781:string)  [unwired: 4 out]
                        n507 = Concatenate Strings(w777, "\\", w775, w773, w774, w773) -> (w784:string)
                        n508 = String To Path(string=w784) -> (path=w786:path)
                        n509 = Concatenate Strings(w784, w783, w781, "-", w780, ".tdms") -> (w772:string)
                        n510 = Create Folder(path (use dialog)=w786) -> (error out=w785:errorcluster)  [unwired: 2 in, 2 out]
                        n511 = global write "Global 1.vi" "LAB01-2 FILE"(w772) -> ()
                        n512 = call <vilib>:"Clear Errors.vi"("error in (no error)"=w785) -> ()  [unwired: 6 in, 1 out]
                      }
                      frame #1 {
                        (unwired) FALSE
                        n513 = String To Path(string=w796) -> (path=w792:path)
                        n514 = TDMS Open(6:FALSE, 10:T18."create or replace" ("operation (0:open)"), 11:w792) -> (0:w791:errorcluster, 3:→"TDMS LAB01-2":refnum<k34>)  [unwired: 4 in]
                      }
                      frame #2 {
                        n515 = local read "SET LAB01-2"() -> (w802:T5)
                        n516 = local read "TDMS LAB01-2"() -> (w813:refnum<k34>)
                        n517 = Build Array("Testers Name", "Description", "Set Test Cycles", "T-Rise minutes", "T-Rise Deg C") -> (w803:string[])
                        n518 = Unbundle(w802) -> ("NAME"=w801:string, "DESCRIPTION"=w800:string, "CYCLES"=w799:dbl, "T-RISE mins"=w798:dbl, "T-RISE deg C"=w797:dbl)
                        n519 = Number To Decimal String(number=w799) -> (decimal integer string=w812:string)  [unwired: 1 in]
                        n520 = Number To Decimal String(number=w798) -> (decimal integer string=w811:string)  [unwired: 1 in]
                        n521 = Number To Decimal String(number=w797) -> (decimal integer string=w810:string)  [unwired: 1 in]
                        n522 = Build Array(w801, w800, w812, w811, w810) -> (w809:string[])
                        n523 = TDMS Set Properties(5:w809, 7:w803, 11:w813) -> ()  [unwired: 3 in, 4 out]
                      }
                      frame #3 {
                        n524 = local read "DISP LAB01-2"() -> (w815:T4)
                        n525 = Concatenate Strings("LAB01-2  ", w818) -> (w819:string)
                        n526 = Two Button Dialog(message=w819, 1:w816, 2:w817) -> (T button?=w821:bool)
                        n527 = case shown="True" w821 {
                          tunnel: w815 -> [w828 w829]
                          tunnel: [w828 w829] -> w825
                          tunnel: [w827 w830] -> w824
                          tunnel: [w826 w830] -> w823
                          frame False {
                            n528 = Unbundle(w828) -> ("CYCLE"=w827:dbl, "MINS"=w826:dbl)  [unwired: 1 out]
                          }
                          frame True {
                            w830 = 0.0
                          }
                        }
                        n529 = Bundle(cluster=w825, "CYCLE"=w824, "MINS"=w823, "STATUS"="RUN") -> (w814:T4)
                        n530 = local write "DISP LAB01-2"(w814) -> ()
                      }
                      frame #4 {
                        n531 = local read "SIG LAB01-2"() -> (w833:T2)
                        n532 = local read "TEMP START LAB01-2"() -> (w835:cluster{"TL":dbl, "TN":dbl})
                        n533 = Unbundle(w833) -> ("Tmp Live"=w832:dbl, "Tmp Neut"=w831:dbl)  [unwired: 3 out]
                        n534 = Bundle(cluster=w835, "TL"=w832, "TN"=w831) -> (w834:cluster{"TL":dbl, "TN":dbl})
                        n535 = local write "TEMP START LAB01-2"(w834) -> ()
                      }
                    }
                  }
                }
              }
              event "RUN LAB02-1": Value Change {
                n536 = event-data() -> ("NewVal"=w839:bool)  [unwired: 1 in, 5 out]
                n537 = local write "run lab02-1"(w839) -> ()
                n538 = case shown="True" w839 {
                  tunnel: w845 -> [_ w881]
                  tunnel: w844 -> [_ w880]
                  tunnel: w842 -> [w847 w879]
                  tunnel: w843 -> [_ w878]
                  tunnel: w841 -> [_ w877]
                  tunnel: [w846 w876] -> w840
                  tunnel: w838 -> [_ w875]
                  tunnel: w837 -> [_ w874]
                  tunnel: w836 -> [_ w873]
                  frame False {
                    # "stop test"
                    n539 = stacked-sequence {
                      tunnel: w847 -> [w856 _]
                      tunnel: [w848 _] -> w846
                      frame #0 {
                        n540 = local read "DISP LAB02-1"() -> (w855:T4)
                        n541 = Unbundle(w855) -> ("CYCLE"=w853:dbl, "MINS"=w854:dbl)  [unwired: 1 out]
                        n542 = case shown="\"CYCLE TEST\"" w856 {
                          tunnel: w854 -> [_ _ w863]
                          tunnel: w853 -> [w861 w862 _]
                          tunnel: [w861 w862 w863] -> w852
                          frame "CHART TEST", Default {
                          }
                          frame "CYCLE TEST" {
                          }
                          frame "T-RISE TEST" {
                          }
                        }
                        n543 = local read "TDMS LAB02-1"() -> (w860:refnum<k34>)
                        n544 = Build Array("STOPPED") -> (w857:string[])
                        n545 = Build Array(w852) -> (w851:dbl[])
                        n546 = TDMS Write(0:w860, 5:"TEST RESULT", 7:w857, 9:w851) -> (4:w849:refnum<k34>, 15:w850:errorcluster)  [unwired: 2 in, 2 out]
                        n547 = TDMS Close(8:w850, 11:w849) -> (0:w848:errorcluster)  [unwired: 1 out]
                      }
                      frame #1 {
                        n548 = local read "DISP LAB02-1"() -> (w867:T4)
                        n549 = stacked-sequence {
                          tunnel: "LAB02-1" -> [w869 w871]
                          frame #0 {
                            n550 = call "sub vi - defrag tdms v1.vi"("panel id"=w869) -> ("error out"=w868:errorcluster)  [unwired: 10 in]
                            n551 = local write "data file error"(w868) -> ()
                          }
                          frame #1 {
                            n552 = local write "RESULT LAB02-1"(FALSE) -> ()
                            n553 = call "Save data file to network drive v2.vi"("panel id"=w871) -> ("network file save error"=w870:errorcluster)  [unwired: 9 in, 1 out]
                            n554 = local write "data file error"(w870) -> ()
                          }
                        }
                        n555 = Bundle(cluster=w867, "STATUS"="STOP") -> (w865:T4)  [unwired: 2 in]
                        n556 = local write "DISP LAB02-1"(w865) -> ()
                      }
                    }
                  }
                  frame True {
                    # "start new test and create test file"
                    n557 = stacked-sequence {
                      seq-local: [w882 _ _ _ _] -> [_ w906 _ _ _]
                      tunnel: w881 -> [w887 _ _ _ _]
                      tunnel: w880 -> [w884 _ _ _ _]
                      tunnel: w879 -> [w897 _ _ _ _]
                      tunnel: w878 -> [w890 _ _ _ _]
                      tunnel: w877 -> [w885 _ _ _ _]
                      tunnel: [_ w901 _ _ _] -> w876
                      tunnel: w875 -> [_ _ _ w927 _]
                      tunnel: w874 -> [_ _ _ w926 _]
                      tunnel: w873 -> [_ _ _ w925 _]
                      frame #0 {
                        w883 = "\\"
                        n558 = local read "SET LAB02-1"() -> (w892:T5)
                        n559 = case shown="\"CYCLE TEST\"" w897 {
                          tunnel: ["L02-1-CHART TEST-" "L02-1-CYCLE TEST-" "L02-1-T-RISE TEST-"] -> w893
                          frame "CHART TEST", Default {
                          }
                          frame "CYCLE TEST" {
                          }
                          frame "T-RISE TEST" {
                          }
                        }
                        n560 = Unbundle(w892) -> ("DESCRIPTION"=w891:string)  [unwired: 4 out]
                        n561 = Concatenate Strings(w887, "\\", w885, w883, w884, w883) -> (w894:string)
                        n562 = String To Path(string=w894) -> (path=w896:path)
